vi "UDP3READ.vi"(0 "Frequency, in Hz":dbl) -> ()   [LabVIEW 2009]
doc: "Reads a UDP stream over channel 1338 (which should be comeing from UDP3LOOP.vi) which sends a flattened variant of the strict type def UDP3.ctl. This function restores this flattened string to the original shape (that of UDP3.ctl) and then passes it to the global variable (global on the rt processor anyway) UDP3rtglob.vi which can be read by outside functions. It's loop can be stopped by setting UDP3rtglob.vi.stop to true, in the same way it's sister function UDP3LOOP.vi is stopped using UDP3GLOB.vi.stop. Frequency is set via an input, and is implemented via quantized wait for ms multiple. The division is preformed only once."
uses:
  UDP 3.ctl
  UDP3rtglob.vi
panel:
  out "Heartbeat":bool
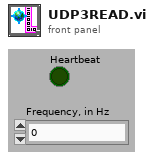
[diagram p1: front panel]
types:
  T1 = typedef "UDP 3.ctl" = cluster{"GPS":cluster{"Lat":dbl, "Longe":dbl}, "INS":cluster{"Heading":dbl, "x-magnetic":dbl, "y-magnetic":dbl, "z-magnetic":dbl, "x-acceleration":dbl, "y-acceleration":dbl, "z-acceleration":dbl}}
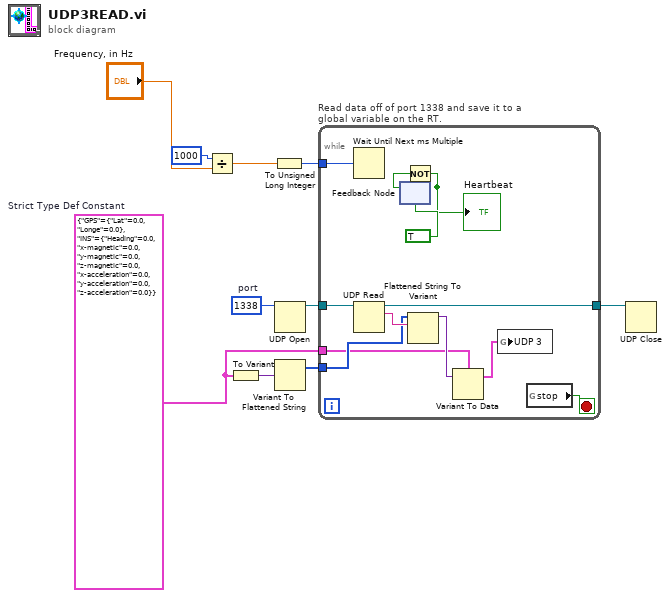
[diagram p0: block diagram]
diagram:
  w5 = T1 {"GPS"={"Lat"=0.0, "Longe"=0.0}, "INS"={"Heading"=0.0, "x-magnetic"=0.0, "y-magnetic"=0.0, "z-magnetic"=0.0, "x-acceleration"=0.0, "y-acceleration"=0.0, "z-acceleration"=0.0}}  # Strict Type Def Constant
  w8 = u16 1338  # port
  n1 = Divide(x=1000, y="Frequency, in Hz") -> (x/y=w2:dbl)
  n2 = To Variant(anything=w5) -> (Variant=w7:variant)
  n3 = To Unsigned Long Integer(number=w2) -> (unsigned 32bit integer=w1:u32)
  n4 = UDP Open(11:w8) -> (port=w9:refnum<k16>)  [unwired: 4 in, 2 out]
  n5 = Variant To Flattened String(Variant=w7) -> (1:w6:i16[])  [unwired: 1 out]
  n6 = while "Read data off of port 1338 and save it to a global variable on the RT." {
    tunnel: [w22] -> w10
    tunnel: w9 -> [w21]
    tunnel: w6 -> [w18]
    tunnel: w5 -> [w17]
    tunnel: w1 -> [w14]
    stop <- w15 stop-if-true
    n7 = Wait Until Next ms Multiple(millisecond multiple=w14) -> ()  [unwired: 1 out]
    n8 = UDP Read(connection ID=w21) -> (data out=w20:string, 3:w22:refnum<k16>)  [unwired: 3 in, 3 out]
    n9 = feedback #1(TRUE) -> (w12:bool)
    n10 = Not(x=w12) -> (.not. x?=w11:bool)
    "Heartbeat" <- w11
    n11 = Flattened String To Variant(6:w20, 7:w18) -> (3:w19:variant)  [unwired: 1 in, 1 out]
    n12 = Variant To Data(Variant=w19, type=w17) -> (data=w16:T1)  [unwired: 1 in, 1 out]
    n13 = global write "UDP3rtglob.vi" "UDP 3"(w16) -> ()
    n14 = global read "UDP3rtglob.vi" "stop"() -> (w15:bool)
  }
  n15 = UDP Close(connection ID=w10) -> ()  [unwired: 1 in, 2 out]
